vi "Daten zu PC.vi"   [LabVIEW 2020, in "Kommunikation mit PC.lvlib"]
uses:
  Kommunikation mit PC.lvlib
  Betriebsstundenzaehler/FGV BSZ Aktionen.ctl
  Regler/Druckregler/Aktionen Param. Druckregler.ctl
  Stickstoff Befuellung/Aktionen Stockstoff Befuellung.ctl
  Verwaltung/FGV IN Aktionen.ctl
  Stoermeldungen/FGV Stoerungen Aktionen.ctl
  Verwaltung/FGV OUT Aktionen.ctl
  Allgemein/FGV Zustaende Aktionen.ctl
  Regler/FGV Daten Regler Aktionen.ctl
  Betriebsstundenzaehler/Betriebsstundenzaehler.lvlib
  Stickstoff Befuellung/Stickstoff Befuellung.lvlib
  Regler/Druckregler/Druckregler.lvlib
  Allgemein/Allgemein.lvlib
  Verwaltung/Verwaltung - cRIO.lvlib
  Stoermeldungen/Stoermeldungen.lvlib
  Regler/Regler.lvlib
  <vilib>/NI_Real-Time Target Support.lvlib
  Externe Stickstoff Befuellung/Externe Stickstoff Befuellung.lvlib
  Externe Stickstoff Befuellung/Aktionen Externe Stockstoff Befuellung.ctl
  CAN Interface/CAN Interface.lvlib
  CAN Interface/FGV CAN Daten Aktionen.ctl
types:
  T1 = typedef "Allgemein.lvlib/FGV Zustaende Aktionen.ctl" = enum16{"lesen", "Zustand PC", "Zustand cRIO", "Bildnummer", "Samplepoint", "Sysloglevel"}
  T2 = typedef "Verwaltung - cRIO.lvlib/FGV OUT Aktionen.ctl" = enum16{"lesen", "ANA OUT", "DO 0-31", "DO 32-47"}
  T3 = typedef "Stoermeldungen.lvlib/FGV Stoerungen Aktionen.ctl" = enum16{"lesen", "Störung aktiv?", "1-64", "65-128"}
  T4 = typedef "Verwaltung - cRIO.lvlib/FGV IN Aktionen.ctl" = enum16{"lesen", "DI", "AI", "Fühler Br.", "TC", "Fühler Br. TC"}
  T5 = typedef "Stickstoff Befuellung.lvlib/Aktionen Stockstoff Befuellung.ctl" = enum16{"lesen", "Befüllen vorbereiten", "Befüllen", "Befüllen beenden", "Warten", "deaktiviert", "initialisieren", "anstehender Fehler"}
  T6 = typedef "Regler.lvlib/Druckregler.lvlib/Aktionen Param. Druckregler.ctl" = enum16{"lesen", "schreiben", "Regler FT-IR", "Regler Ausgang", "Regler Durchfluss", "Regler PMA", "Regler NDIR", "Regler Filterblock", "Regler Gaskühler", "Regler Kalter Block"}
  T7 = typedef "Betriebsstundenzaehler.lvlib/FGV BSZ Aktionen.ctl" = enum16{"Lesen", "Initialisieren", "Starten Pumpe", "Zählen Pumpe", "Starten FT-IR", "Zählen FT-IR"}
  T8 = typedef "CAN Interface.lvlib/FGV CAN Daten Aktionen.ctl" = enum16{"lesen", "Daten", "Konfig", "laden", "speichern", "Status"}
  T9 = typedef "Externe Stickstoff Befuellung.lvlib/Aktionen Externe Stockstoff Befuellung.ctl" = enum16{"lesen", "Befüllen vorbereiten", "Befüllen", "Befüllen beenden", "Warten", "deaktiviert", "initialisieren"}
  T10 = typedef "Regler.lvlib/FGV Daten Regler Aktionen.ctl" = enum16{"lesen", "Out%", "Heizung EIN"}
  T11 = typedef "Bildwechsel.lvlib/Bild-Auswahl.ctl" = enum16{"lesen", "Initialisieren", "Beenden", "Grafik", "Anlagenübersicht", "Anlagengrenzwerte", "Log Konfig", "Gaszuordnung AO", "Erw. Konfiguration", "FT-IR  ", "Störmeldungen", "Störmeldepuffer", "Störmeldekonfig", "PNS Grenzwerte", "Statusübersicht", "Linearisierung", "ARN", "EPA Dichtheitstest", "FID", "PMA", "CalGas", "Lambda", "Interference", "Amium PNS", "EPA T90", "Interference N2O", "Scheduler", "Systemeinstellungen", "EPA Drift", "CAN Konfig"}
  T12 = typedef "Funktionstasten.lvlib/Zustaende.ctl" = enum16{"Standby", "Pause", "Eco", "Messen", "Kalibrieren", "Spülen Filter", "Spülen Leitung", "Umgebungsluft", "0-Gas", "Cal-Gas", "CG zu PNS", "-------------", "Init 1", "Init 2", "Init 3", "Init 4", "Messen vorbereiten", "Messen durchführen", "Exit"}
  T13 = typedef "Verwaltung - cRIO.lvlib/Digital Eingaenge 0-15.ctl" = cluster{"I0: N2 Nachf. FT-IR voll":bool, "I1: N2 Nachf. Vorrat leer":bool, "I2: (Klimaanlage eingeschaltet)":bool, "I3: (Klimaanlage Störung)":bool, "I4: Trigger Eingang (Messdaten sp.)":bool, "I5: Reserve":bool, "I6: Reserve":bool, "I7: Reserve":bool, "I8: Druckschalter Versorgung ok":bool, "I9: Reserve":bool, "I10: Reserve":bool, "I11: Reserve":bool, "I12: Drucksch. N2 Versorgung":bool, "I13: Reserve":bool, "I14: Drucksch. N2 Optikbox":bool, "I15: (Füllstand Kondensatbehälter)":bool}
  T14 = typedef "Verwaltung - cRIO.lvlib/Analog Eingaenge.ctl" = cluster{"AI0: Durchfluss FT-IR":sgl, "AI1: Druck Ausgang":sgl, "AI2: Umgebungsdruck":sgl, "AI3: Druck FT-IR":sgl, "AI4: Druck CalGas":sgl, "AI5: Reserve":sgl, "AI6: Reserve":sgl, "AI7: Reserve":sgl, "Rohwert Durchfluss FT-IR":sgl, "Rohwert Druck Ausgang":sgl, "Rohwert Umgebungsdruck":sgl, "Rohwert Druck FT-IR":sgl, "Rohwert Druck CalGas":sgl, "Rohwert AI5":sgl, "Rohwert AI6":sgl, "Rohwert AI7":sgl, "Rohwert Diffdruck mbar FTIR":sgl}
  T15 = typedef "Verwaltung - cRIO.lvlib/TC Eingaenge.ctl" = cluster{"TC0: Reserve":sgl, "TC1: HL zu FT-IR":sgl, "TC2: HL Extern SP1":sgl, "TC3: HL Extern SP2":sgl, "TC4: Reserve":sgl, "TC5: Reserve":sgl, "TC6: Reserve":sgl, "TC7: Reserve":sgl, "TC8: FT-IR":sgl, "TC9: Reserve":sgl, "TC10: Schaltschrank":sgl, "TC11: Umgebung":sgl}
  T16 = typedef "Verwaltung - cRIO.lvlib/Digital Ausgaenge 32-63.ctl" = cluster{"O32: Messgaspumpe EIN":bool, "O33: (Umgebungsluftpumpe)":bool, "O34: (Kondensatpumpe GK)":bool, "O35: Klima/Lüfter EIN":bool, "O36: Versorgung Heizungen":bool, "O37: Versorgung Heizungen":bool, "O38: (Gaskühler EIN (Freigabe))":bool, "O39: Störung FAS LP":bool, "O40: (Heizung Filterblock)":bool, "O41: Heizung HL zu FT-IR":bool, "O42: Heizung HL Extern SP1":bool, "O43: Heizung HL Extern SP2":bool, "O44: Heizung Reserve":bool, "O45: Heizung Reserve":bool, "O46: Statusbeleuchtung grün":bool, "O47: Statusbeleuchtung rot":bool}
  T17 = typedef "Verwaltung - cRIO.lvlib/Digital Ausgaenge 0-31.ctl" = cluster{"O0: Druckluft Versorgung":bool, "O1: CG 1 (FB Eingang 1)":bool, "O2: CG 2 (Kühlung FT-IR EIN)":bool, "O3: CG 3 (FB Bypass)":bool, "O4: CG 4 (FB CalGas)":bool, "O5: CG 5 (FB spülen/UL)":bool, "O6: CG 6 (FB zum FT-IR)":bool, "O7: CG 7 (FB zum FID)":bool, "O8: CG 8 (FB Reserve)":bool, "O9: (FB Reserve)":bool, "O10: (FB Umgebungsluft FID)":bool, "O11: (FB zum Gaskühler)":bool, "O12: FB Stickstoff zu FT-IR":bool, "O13: Optikbox FT-IR spülen":bool, "O14: (Purifier deaktivieren)":bool, "O15: (Umschaltung Purifier/Stickstoff)":bool, "O16: N2 Einblasung":bool, "O17: LSP LN2 Nachfüllung":bool, "O18: (Reserve)":bool, "O19: (Pumpe Eingang1)":bool, "O20: (Pumpe Eingang2)":bool, "O21: (Pumpe Spülen1)":bool, "O22: (Pumpe Spülen2)":bool, "O23: (Reserve)":bool, "O24: CalGas 1":bool, "O25: CalGas 2":bool, "O26: CG 3-8 (CalGas 3)":bool, "O27: Stickstoff aufschalten":bool, "O28: CG zu PNS":bool, "O29: FTIR Standby Spülung":bool, "O30: CG zu Entnahme(T90)":bool, "O31: (Purifier regenerieren)":bool}
  T18 = typedef "NI_Real-Time Target Support.lvlib/RT CPU Load.ctl" = cluster{"Total (%)":dbl, "Time Critical (%)":dbl, "Timed Structures (%)":dbl, "High (%)":dbl, "Above Normal (%)":dbl, "Normal (%)":dbl, "Background (%)":dbl, "Idle (%)":dbl, "ISR (%)":dbl}
  T19 = cluster{"Total (%)":sgl, "Time Critical (%)":sgl, "Timed Structures (%)":sgl, "High (%)":sgl, "Above Normal (%)":sgl, "Normal (%)":sgl, "Background (%)":sgl, "Idle (%)":sgl, "ISR (%)":sgl}
  T20 = cluster{"Output% 1":i16, "Output% 2":i16, "Output% 3":i16, "Output% 4":i16, "Output% 5":i16, "Output% 6":i16, "Output% 7":i16, "Output% 8":i16, "Output% 9":i16, "Output% 10":i16, "Output% 11":i16, "Output% 12":i16, "Output% 13":i16, "Output% 14":i16, "Output% 15":i16, "Output% 16":i16, "Output% 17":i16, "Output% 18":i16}
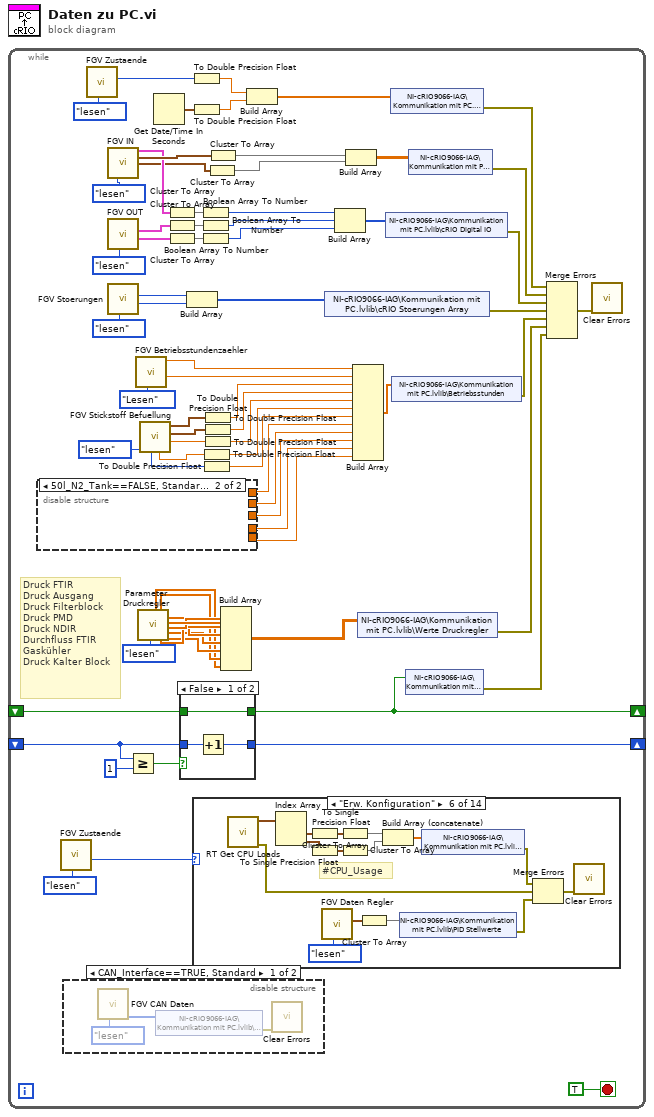
[diagram p0: block diagram]
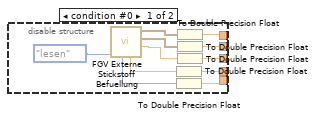
[diagram p3: hidden frame]
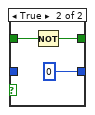
[diagram p17: hidden frame]
diagram:
  n1 = while {
    shift-right: [w49] -> _
    shift-left: _ -> [w50]
    shift-right: [w52] -> _
    shift-left: _ -> [w51]
    stop <- TRUE stop-if-true
    # "Druck FTIR\nDruck Ausgang\nDruck Filterblock\nDruck PMD\nDruck NDIR\nDurchfluss FTIR\nGaskühler\nDruck Kalter Block"
    n2 = disable-structure shown="50l_N2_Tank==FALSE, Standard" {
      disable-tunnel: [w82 _] -> w5
      disable-tunnel: [w81 _] -> w4
      disable-tunnel: [w80 _] -> w3
      disable-tunnel: [w79 _] -> w2
      disable-tunnel: [w78 _] -> w1
      frame condition #0 {
        n3 = call "FGV Externe Stickstoff Befuellung.vi"("Aktion"=Aktionen_Externe_Stockstoff_Befuellung."lesen") -> ("Befülldauer"=w85:sgl, "Befüllen 2"=w86:timestamp, "Befüllen 1"=w87:timestamp, "Befüllzeit"=w84:dbl, "Aktion"=w83:T9)  [unwired: 4 in, 2 out]
        n4 = To Double Precision Float(number=w84) -> (double precision float=w79:dbl)
        n5 = To Double Precision Float(number=w83) -> (double precision float=w78:dbl)
        n6 = To Double Precision Float(number=w87) -> (double precision float=w82:dbl)
        n7 = To Double Precision Float(number=w86) -> (double precision float=w81:dbl)
        n8 = To Double Precision Float(number=w85) -> (double precision float=w80:dbl)
      }
      frame condition #1 (active) {
      }
    }
    n9 = call "FGV Zustaende.vi"("Aktionen"=FGV_Zustaende_Aktionen."lesen") -> ("aktuelle Bildnummer"=w26:T11)  [unwired: 6 in, 4 out]
    n10 = disable-structure shown="CAN_Interface==TRUE, Standard" {
      frame condition #0 {
        n11 = call "FGV CAN Daten.vi"("Aktionen"=FGV_CAN_Daten_Aktionen."lesen") -> ("Status"=w76:u32[])  [unwired: 8 in, 2 out]
        n12 = shared-variable "NI-cRIO9066-IAG\\Kommunikation mit PC.lvlib\\CAN_Status"(w76) -> (error out=w75:errorcluster)  [unwired: 1 in]
        n13 = call <vilib>:"Clear Errors.vi"("error in (no error)"=w75) -> ()  [unwired: 5 in, 2 out]
      }
      frame condition #1 (active) {
      }
    }
    n14 = call "FGV Zustaende.vi"("Aktionen"=FGV_Zustaende_Aktionen."lesen") -> ("Zustand cRIO"=w37:T12)  [unwired: 6 in, 4 out]
    n15 = call "FGV IN.vi"("Aktion"=FGV_IN_Aktionen."lesen") -> ("DI"=w31:T13, "Analog Eingänge"=w35:T14, "TC Eingänge"=w19:T15)  [unwired: 10 in, 2 out]
    n16 = call "FGV OUT.vi"("Aktion"=FGV_OUT_Aktionen."lesen") -> ("DO 32-63"=w28:T16, "DO 0-31"=w29:T17)  [unwired: 7 in, 2 out]
    n17 = call "FGV Stoerungen.vi"("Aktionen"=FGV_Stoerungen_Aktionen."lesen") -> ("65-128"=w32:u64, "1-64"=w33:u64)  [unwired: 8 in, 1 out]
    n18 = Greater Or Equal?(x=w51, y=u16 1) -> (x >= y?=w54:bool)
    n19 = call "FGV Betriebsstundenzaehler.vi"("BSZ Aktionen"=FGV_BSZ_Aktionen."Lesen") -> ("Betriebsstunden FT-IR"=w67:dbl, "Betriebsstunden Pumpe"=w68:dbl)  [unwired: 9 in]
    n20 = call "Parameter Druckregler.vi"("Aktionen"=Aktionen_Param._Druckregler."lesen") -> ("Werte Kalter Block"=w10:sgl[], "Werte Gaskühler"=w11:sgl[], "Werte Filterblock"=w15:sgl[], "Werte PMA"=w14:sgl[], "Werte FT-IR"=w17:sgl[], "Werte Ausgang"=w16:sgl[], "Werte NDIR"=w13:sgl[], "Werte Durchfluss"=w12:sgl[])  [unwired: 10 in, 1 out]
    n21 = call "FGV Stickstoff Befuellung.vi"("Aktion"=Aktionen_Stockstoff_Befuellung."lesen") -> ("Befülldauer"=w39:sgl, "Befüllen 2"=w40:timestamp, "Befüllen 1"=w41:timestamp, "Warten/Befüllzeit"=w9:dbl, "Aktion"=w7:T5)  [unwired: 4 in, 2 out]
    n22 = Get Date/Time In Seconds() -> (seconds since 1Jan1904=w66:timestamp)
    n23 = Cluster To Array(cluster=w31) -> (array=w74:bool[])
    n24 = Cluster To Array(cluster=w29) -> (array=w73:bool[])
    n25 = Cluster To Array(cluster=w28) -> (array=w62:bool[])
    n26 = case shown="False" w54 {
      tunnel: [w106 u16 0] -> w52
      tunnel: w51 -> [w105 _]
      tunnel: [w104 w108] -> w49
      tunnel: w50 -> [w104 w107]
      frame False {
        n27 = Increment(x=w105) -> (x+1=w106:u16)
      }
      frame True {
        n28 = Not(x=w107) -> (.not. x?=w108:bool)
      }
    }
    n29 = Build Array(w33, w32) -> (w23:u64[])
    n30 = To Double Precision Float(number=w37) -> (double precision float=w64:dbl)
    n31 = To Double Precision Float(number=w66) -> (double precision float=w65:dbl)
    n32 = case shown="\"Erw. Konfiguration\"" w26 {
      frame "Grafik", Default {
      }
      frame "Anlagenübersicht" {
      }
      frame "Anlagengrenzwerte" {
      }
      frame "Log Konfig" {
      }
      frame "Gaszuordnung AO" {
      }
      frame "Erw. Konfiguration" {
        # "#CPU_Usage"
        n33 = call <vilib>:"RT Get CPU Loads.vi"() -> ("error out"=w93:errorcluster, "CPU loads"=w96:T18[])  [unwired: 10 in]
        n34 = Index Array(array=w96) -> (element #1=w95:T18, element #2=w89:T18)  [unwired: 2 in]
        n35 = To Single Precision Float(number=w95) -> (single precision float=w91:T19)
        n36 = To Single Precision Float(number=w89) -> (single precision float=w92:T19)
        n37 = call "FGV Daten Regler.vi"("Aktionen"=FGV_Daten_Regler_Aktionen."lesen") -> ("PID - OUT%"=w97:T20)  [unwired: 9 in, 1 out]
        n38 = Cluster To Array(cluster=w91) -> (array=w103:sgl[])
        n39 = Cluster To Array(cluster=w92) -> (array=w90:sgl[])
        n40 = Cluster To Array(cluster=w97) -> (array=w101:i16[])
        n41 = Build Array (concatenate)(w103, w90) -> (w102:sgl[])
        n42 = shared-variable "NI-cRIO9066-IAG\\Kommunikation mit PC.lvlib\\PID Stellwerte"(w101) -> (error out=w99:errorcluster)  [unwired: 1 in]
        n43 = shared-variable "NI-cRIO9066-IAG\\Kommunikation mit PC.lvlib\\CPU Status"(w102) -> (error out=w94:errorcluster)  [unwired: 1 in]
        n44 = Merge Errors(w94, w93, w99) -> (w100:errorcluster)
        n45 = call <vilib>:"Clear Errors.vi"("error in (no error)"=w100) -> ()  [unwired: 5 in, 2 out]
      }
      frame "FT-IR  " {
      }
      frame "Initialisieren" {
      }
      frame "Beenden" {
      }
      frame "lesen" {
      }
      frame "PNS Grenzwerte" {
      }
      frame "Störmeldungen" {
      }
      frame "Störmeldepuffer" {
      }
      frame "Störmeldekonfig" {
      }
    }
    n46 = Boolean Array To Number(Boolean array=w74) -> (number=w72:u32)
    n47 = Boolean Array To Number(Boolean array=w73) -> (number=w71:u32)
    n48 = Boolean Array To Number(Boolean array=w62) -> (number=w61:u32)
    n49 = To Double Precision Float(number=w9) -> (double precision float=w8:dbl)
    n50 = To Double Precision Float(number=w7) -> (double precision float=w6:dbl)
    n51 = To Double Precision Float(number=w41) -> (double precision float=w59:dbl)
    n52 = To Double Precision Float(number=w40) -> (double precision float=w58:dbl)
    n53 = To Double Precision Float(number=w39) -> (double precision float=w57:dbl)
    n54 = Cluster To Array(cluster=w19) -> (array=w20:sgl[])
    n55 = Cluster To Array(cluster=w35) -> (array=w21:sgl[])
    n56 = Build Array(w17, w16, w15, w14, w13, w12, w11, w10) -> (w48:sgl[][])
    n57 = Build Array(w64, w65) -> (w63:dbl[])
    n58 = shared-variable "NI-cRIO9066-IAG\\Kommunikation mit PC.lvlib\\cRIO Stoerungen Array"(w23) -> (error out=w22:errorcluster)  [unwired: 1 in]
    n59 = Build Array(w72, w71, w61) -> (w70:u32[])
    n60 = Build Array(w21, w20) -> (w18:sgl[][])
    n61 = Build Array(w68, w67, w59, w58, w57, w8, w6, w5, w4, w3, w2, w1) -> (w60:dbl[])
    n62 = shared-variable "NI-cRIO9066-IAG\\Kommunikation mit PC.lvlib\\Werte Druckregler"(w48) -> (error out=w44:errorcluster)  [unwired: 1 in]
    n63 = shared-variable "NI-cRIO9066-IAG\\Kommunikation mit PC.lvlib\\cRIO Digital IO"(w70) -> (error out=w27:errorcluster)  [unwired: 1 in]
    n64 = shared-variable "NI-cRIO9066-IAG\\Kommunikation mit PC.lvlib\\cRIO lebt"(w63) -> (error out=w47:errorcluster)  [unwired: 1 out]
    n65 = shared-variable "NI-cRIO9066-IAG\\Kommunikation mit PC.lvlib\\Betriebsstunden"(w60) -> (error out=w45:errorcluster)  [unwired: 1 in]
    n66 = shared-variable "NI-cRIO9066-IAG\\Kommunikation mit PC.lvlib\\LifeBit"(w49) -> (error out=w24:errorcluster)  [unwired: 1 in]
    n67 = shared-variable "NI-cRIO9066-IAG\\Kommunikation mit PC.lvlib\\cRIO AI"(w18) -> (error out=w46:errorcluster)  [unwired: 1 out]
    n68 = Merge Errors(w47, w46, w27, w22, w45, w44, w24) -> (w43:errorcluster)
    n69 = call <vilib>:"Clear Errors.vi"("error in (no error)"=w43) -> ()  [unwired: 5 in, 2 out]
  }
